vi "FPGA tester.vi"() -> ()   [LabVIEW 2014]
uses:
  <instrlib>/ni272xReferenceVIs/ni272xReferenceVIs.llb/ni272x Connector Identifier.ctl
  <instrlib>/ni272xReferenceVIs/ni272xReferenceVIs.llb/ni272x Write Resistance 1Chan 1Samp.vi
  <instrlib>/ni272xReferenceVIs/ni272xReferenceVIs.llb/ni272x Connect to Connector 1Chan.vi
  <vilib>/FPGAPlugInAG/PXI-7854R/niLvFpga_Open_PXI-7854R.vi
  <vilib>/rvi/interface/common/dynamic/niFpgaDynamicAddResources.vi
  <vilib>/Utility/error.llb/Error Cluster From Error Code.vi
  <vilib>/rvi/errors/niLvFpgaAdjustHostInterfaceError.vi
  <vilib>/rvi/interface/nirviOpenFPGA/nirviOpenFPGA.xnode
  FPGA Bitfiles/UEGOSimCustomDev_FPGATarget_examplefpgacode_CnYhSZw3IHk.lvbitx
  FPGA/example fpga code.vi
  <vilib>/rvi/interface/nirviReadWriteControl/nirviReadWriteControl.xnode
  NiFpgaLv.dll
  <vilib>/rvi/interface/Simulation/niFpgaSimulationCallBeginRW.vi
panel:
  in  "DAQmx Device Name":tag="PXI1Slot8"
  in  "Resistance Requested":dbl
  out "coerced resistance (ohms)":dbl
  out "PWM ADC count":i16
  in  "Stop Button":bool
  out "Waveform Chart":cluster{"PWM low time":u32, "PWM high time":u32}(graph)
  out "UEGO.1.in":cluster{"PWM low time":u32, "PWM high time":u32}
  in  "UEGO.1.out":T1={"Sensor Model"=enum."Bosch 4.2", "lambda"=1.0, "cal"=FALSE, "negate"=FALSE, "PWM threshold"=-15000, "PWM timeout"=40000000} {"lambda" format="%.10g"}
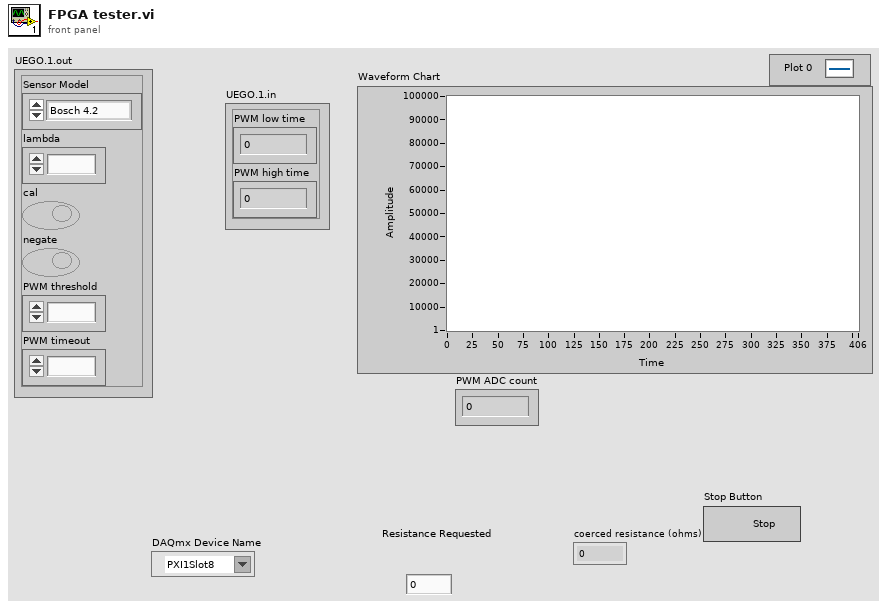
[diagram p1: front panel]
types:
  T1 = cluster{"Sensor Model":enum16{"Narrow Band", "Bosch 4.2", "Bosch 4.9"}, "lambda":fxp<+,12,3>, "cal":bool, "negate":bool, "PWM threshold":i16, "PWM timeout":u32}
  T2 = enum16{"open", "open or create", "create or replace", "create", "open (read-only)"}
  T3 = typedef "ni272x Reference.ctl" = refnum<k20>
  T4 = typedef "ni272x Connector Identifier.ctl" = enum8{"DUT Connector", "DMM Test Connector"}
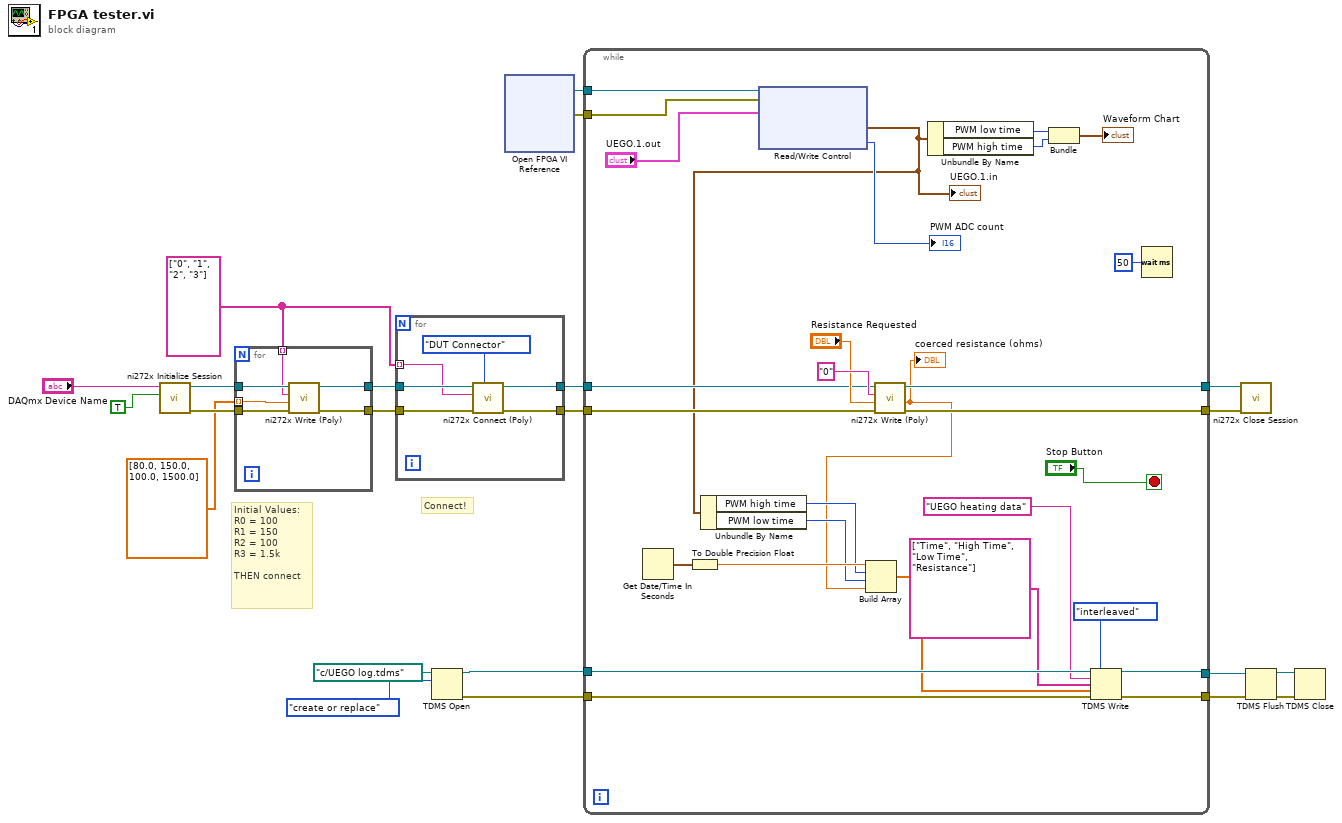
[diagram p0: block diagram]
diagram:
  w13 = string[] ["0", "1", "2", "3"]
  # "Connect!"
  # "Initial Values:\nR0 = 100\nR1 = 150\nR2 = 100\nR3 = 1.5k\n\nTHEN connect"
  n1 = call <instrlib>:"ni272x Initialize Session.vi"("reset device (T)"=TRUE, "DAQmx Device Name"="DAQmx Device Name") -> ("error out"=w15:errorcluster, "instrument handle out"=w18:T3)  [unwired: 8 in]
  n2 = for {
    tunnel: w18 -> [w28]
    tunnel: [w27] -> w17
    tunnel: [w26] -> w16
    tunnel: w15 -> [w25]
    tunnel: w13 -> [w24] mode=indexing
    tunnel: dbl[] [80.0, 150.0, 100.0, 1500.0] -> [w23] mode=indexing
    n3 = call-poly <instrlib>:"ni272x Write (Poly).vi"("error in (no error)"=w25, "requested resistance (ohms)"=w23, "resistor channel"=w24, "instrument handle"=w28) -> ("error out"=w26:errorcluster, "instrument handle out"=w27:T3)  [unwired: 5 in, 1 out]
  }
  n4 = for {
    tunnel: [w34] -> w11
    tunnel: [w33] -> w12
    tunnel: w17 -> [w31]
    tunnel: w16 -> [w30]
    tunnel: w13 -> [w29] mode=indexing
    n5 = call-poly <instrlib>:"ni272x Connect (Poly).vi"("connector identifier"=ni272x_Connector_Identifier."DUT Connector", "error in (no error)"=w30, "resistor channel"=w29, "instrument handle"=w31) -> ("error out"=w34:errorcluster, "instrument handle out"=w33:T3)  [unwired: 6 in]
  }
  n6 = TDMS Open(10:T2."create or replace" ("operation (0:open)"), 11:path "c:/UEGO log.tdms" ("file path")) -> (0:w7:errorcluster, 3:w8:refnum<k34>)  [unwired: 5 in]
  n7 = xnode "Open FPGA VI Reference"() -> ("FPGA VI Reference Out"=w22:refnum<k20>, "error out"=w21:errorcluster)  [unwired: 2 in]
  n8 = while {
    tunnel: w22 -> [w62]
    tunnel: w21 -> [w61]
    tunnel: w12 -> [w52]
    tunnel: w11 -> [w51]
    tunnel: [w50] -> w10
    tunnel: [w49] -> w9
    tunnel: w8 -> [w48]
    tunnel: w7 -> [w47]
    tunnel: [w46] -> w6
    tunnel: [w45] -> w5
    stop <- "Stop Button" stop-if-true
    n9 = Get Date/Time In Seconds() -> (seconds since 1Jan1904=w43:timestamp)
    n10 = To Double Precision Float(number=w43) -> (double precision float=w42:dbl)
    n11 = xnode "Read/Write Control"("FPGA VI Reference In"=w62, "error in"=w61, "UEGO.1.out"="UEGO.1.out") -> ("UEGO.1.in"=w39:cluster{"PWM low time":u32, "PWM high time":u32}, "PWM ADC count"=→"PWM ADC count":i16)  [unwired: 2 out]
    "UEGO.1.in" <- w39
    n12 = Unbundle By Name(w39) -> ("PWM high time"=w38:u32, "PWM low time"=w37:u32)
    n13 = call-poly <instrlib>:"ni272x Write (Poly).vi"("error in (no error)"=w51, "requested resistance (ohms)"="Resistance Requested", "resistor channel"="0", "instrument handle"=w52) -> ("error out"=w49:errorcluster, "coerced resistance (ohms)"=w36:dbl, "instrument handle out"=w50:T3)  [unwired: 5 in]
    "coerced resistance (ohms)" <- w36
    n14 = Build Array(w42, w38, w37, w36) -> (w44:dbl[])
    n15 = Unbundle By Name(w39) -> ("PWM low time"=w57:u32, "PWM high time"=w56:u32)
    n16 = Bundle("PWM low time"=w57, "PWM high time"=w56) -> (→"Waveform Chart":cluster{"PWM low time":u32, "PWM high time":u32})  [unwired: 1 in]
    n17 = TDMS Write(0:w48, 1:enum16{"decimated", "interleaved"}."interleaved" ("data layout (0:decimated)"), 5:"UEGO heating data" ("group name in (Untitled)"), 7:string[] ["Time", "High Time", "Low Time", "Resistance"] ("channel name(s) in (Untitled)"), 9:w44, 11:w47) -> (4:w46:refnum<k34>, 15:w45:errorcluster)  [unwired: 2 out]
    n18 = Wait (ms)(milliseconds to wait=u32 50) -> ()  [unwired: 1 out]
  }
  n19 = call <instrlib>:"ni272x Close Session.vi"("error in (no error)"=w9, "instrument handle"=w10) -> ()  [unwired: 9 in, 1 out]
  n20 = TDMS Flush(4:w5, 7:w6) -> (0:w4:errorcluster, 3:w3:refnum<k34>)
  n21 = TDMS Close(8:w4, 11:w3) -> ()  [unwired: 2 out]
